vi "Find Main vi path.vi"(8 "error in":errorcluster, 11 "Library Path":path) -> (0 "error out":errorcluster, 2 "Main.vi Found?":bool, 3 "Main vi Path":path)   [LabVIEW 2020, in "Panther Dashboard.lvlib"]
uses:
  Panther Dashboard.lvlib
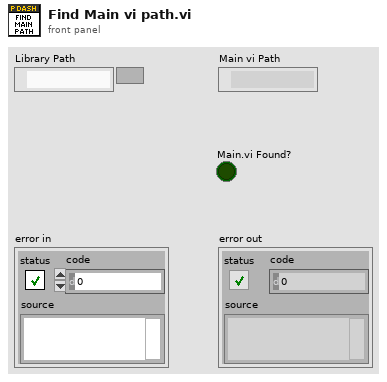
[diagram p1: front panel]
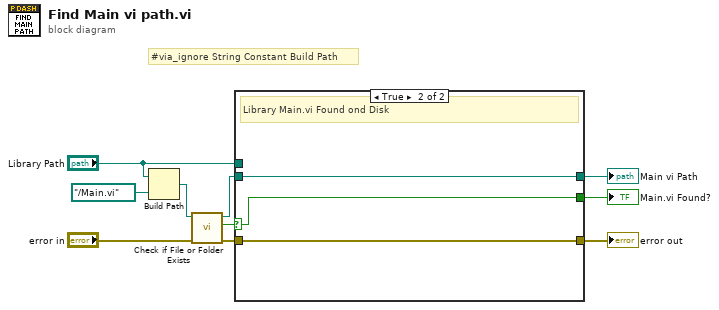
[diagram p0: block diagram]
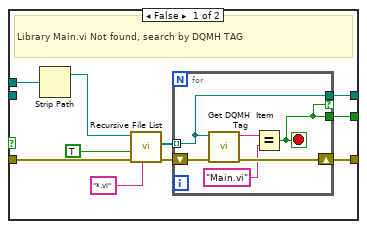
[diagram p2: hidden frame]
diagram:
  # "#via_ignore String Constant Build Path"
  n1 = Build Path(base path="Library Path", name or relative path=path "../Main.vi") -> (appended path=w6:path)
  n2 = call <vilib>:"Check if File or Folder Exists.vi"("error in (no error)"="error in", "path"=w6) -> ("error out"=w10:errorcluster, "file or folder exists?"=w4:bool, "dup path"=w5:path)  [unwired: 7 in]
  n3 = case shown="True" w4 {
    selector: w4 -> [_ w28]
    tunnel: [w20 w29] -> w8
    tunnel: w10 -> [w19 w29]
    tunnel: w5 -> [_ w27]
    tunnel: [w13 w28] -> w2
    tunnel: [w12 w27] -> w3
    tunnel: "Library Path" -> [w11 _]
    frame False {
      # "Library Main.vi Not found, search by DQMH TAG"
      n4 = Strip Path(path=w11) -> (stripped path=w17:path)  [unwired: 1 out]
      n5 = call <vilib>:"Recursive File List.vi"("pattern"="*.vi", "error in (no error)"=w19, "Continue Recursing on Error? (F)"=TRUE, "Folder Path"=w17) -> ("error out"=w18:errorcluster, "All Files in Dir"=w14:path[])  [unwired: 3 in, 3 out]
      n6 = for {
        shift-right: [w25] -> w20
        shift-left: w18 -> [w26]
        tunnel: w14 -> [w22] mode=indexing
        tunnel: [w21] -> w13
        tunnel: [w22] -> w12 if=w21
        stop <- w21 stop-if-true
        n7 = call "Get DQMH  Item Tag.vi"("error in"=w26, "Path"=w22) -> ("error out"=w25:errorcluster, "DQMH Tag"=w24:string)  [unwired: 8 in]
        n8 = Equal?(x=w24, y="Main.vi") -> (x = y?=w21:bool)
      }
    }
    frame True {
      # "Library Main.vi Found ond Disk"
    }
  }
  "Main vi Path" <- w3
  "Main.vi Found?" <- w2
  "error out" <- w8
